vi "r.vi"() -> ()   [LabVIEW 2013]
panel:
  out "error out 3":errorcluster
  out "error out 2":errorcluster
  out "error out":errorcluster
  out "URL":string
  out "URL Selected":bool
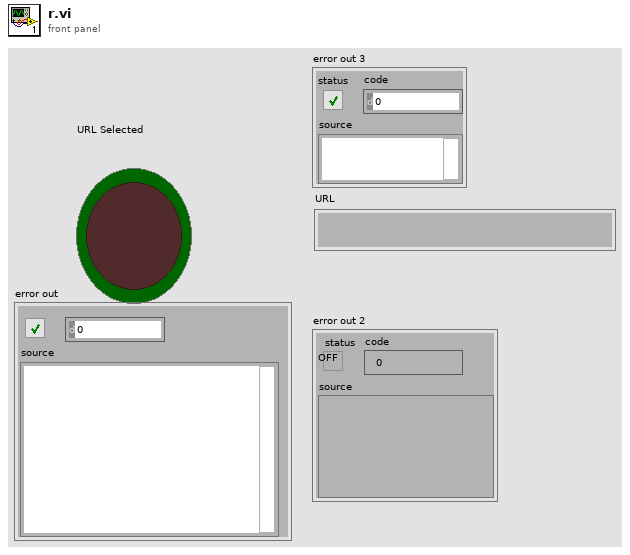
[diagram p1: front panel]
types:
  T1 = enum16{"Read", "Write", "ReadWrite", "BufferedRead", "BufferedReadWrite"}
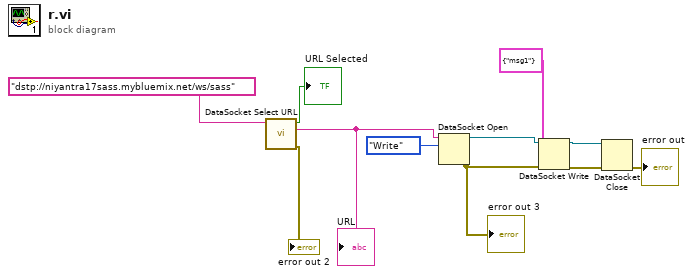
[diagram p0: block diagram]
diagram:
  n1 = call <vilib>:"DataSocket Select URL.vi"("StartURL (empty)"="dstp://niyantra17sass.mybluemix.net/ws/sass") -> ("error out"=→"error out 2":errorcluster, "URL"=w3:string, "URL Selected"=→"URL Selected":bool)  [unwired: 8 in]
  "URL" <- w3
  n2 = DataSocket Open(10:T1."Write" ("mode"), 11:w3) -> (0:w9:errorcluster, 3:w10:refnum<k13>)  [unwired: 2 in]
  "error out 3" <- w9
  n3 = DataSocket Write(8:w9, 10:cluster{string} {"msg1"} ("data"), 11:w10) -> (0:w6:errorcluster, 3:w7:refnum<k13>)  [unwired: 1 in, 1 out]
  n4 = DataSocket Close(8:w6, 11:w7) -> (0:→"error out":errorcluster)  [unwired: 1 in, 1 out]
